vi "DROPBEAR_Model_Updating_Postprocessing.vi"(8 "error in (no error)":errorcluster, 11 "DROPBEAR_Model_Updating in":refnum<class "DROPBEAR_Model_Updating.lvclass">) -> (0 "Cycle time (ms)":dbl, 1 "Signal Quality":T3, 2 "Timing stats":T1, 3 "Plots":T2)   [LabVIEW 2021, in "DROPBEAR_Model_Updating.lvclass"]
uses:
  DROPBEAR_Model_Updating.lvclass
  DROPBEAR_Model_Updating.lvclass/DROPBEAR_Model_Updating.ctl
  Online_TRAC/Online_TRAC.lvclass/Online_TRAC.ctl
  Online_SNR/Online_SNR.lvclass/Online_SNR.ctl
  Read Distributional Statistics.vi
  Data_Array/Data_Array.lvclass
  Online_Statistic/Online_Statistic.lvclass
  Online_SNR/Online_SNR.lvclass
  Online_TRAC/Online_TRAC.lvclass
panel:
  out "Frequency":dynamicdata(graph)
  out "Nodal":dynamicdata(graph)
  out "Meter":dynamicdata(graph)
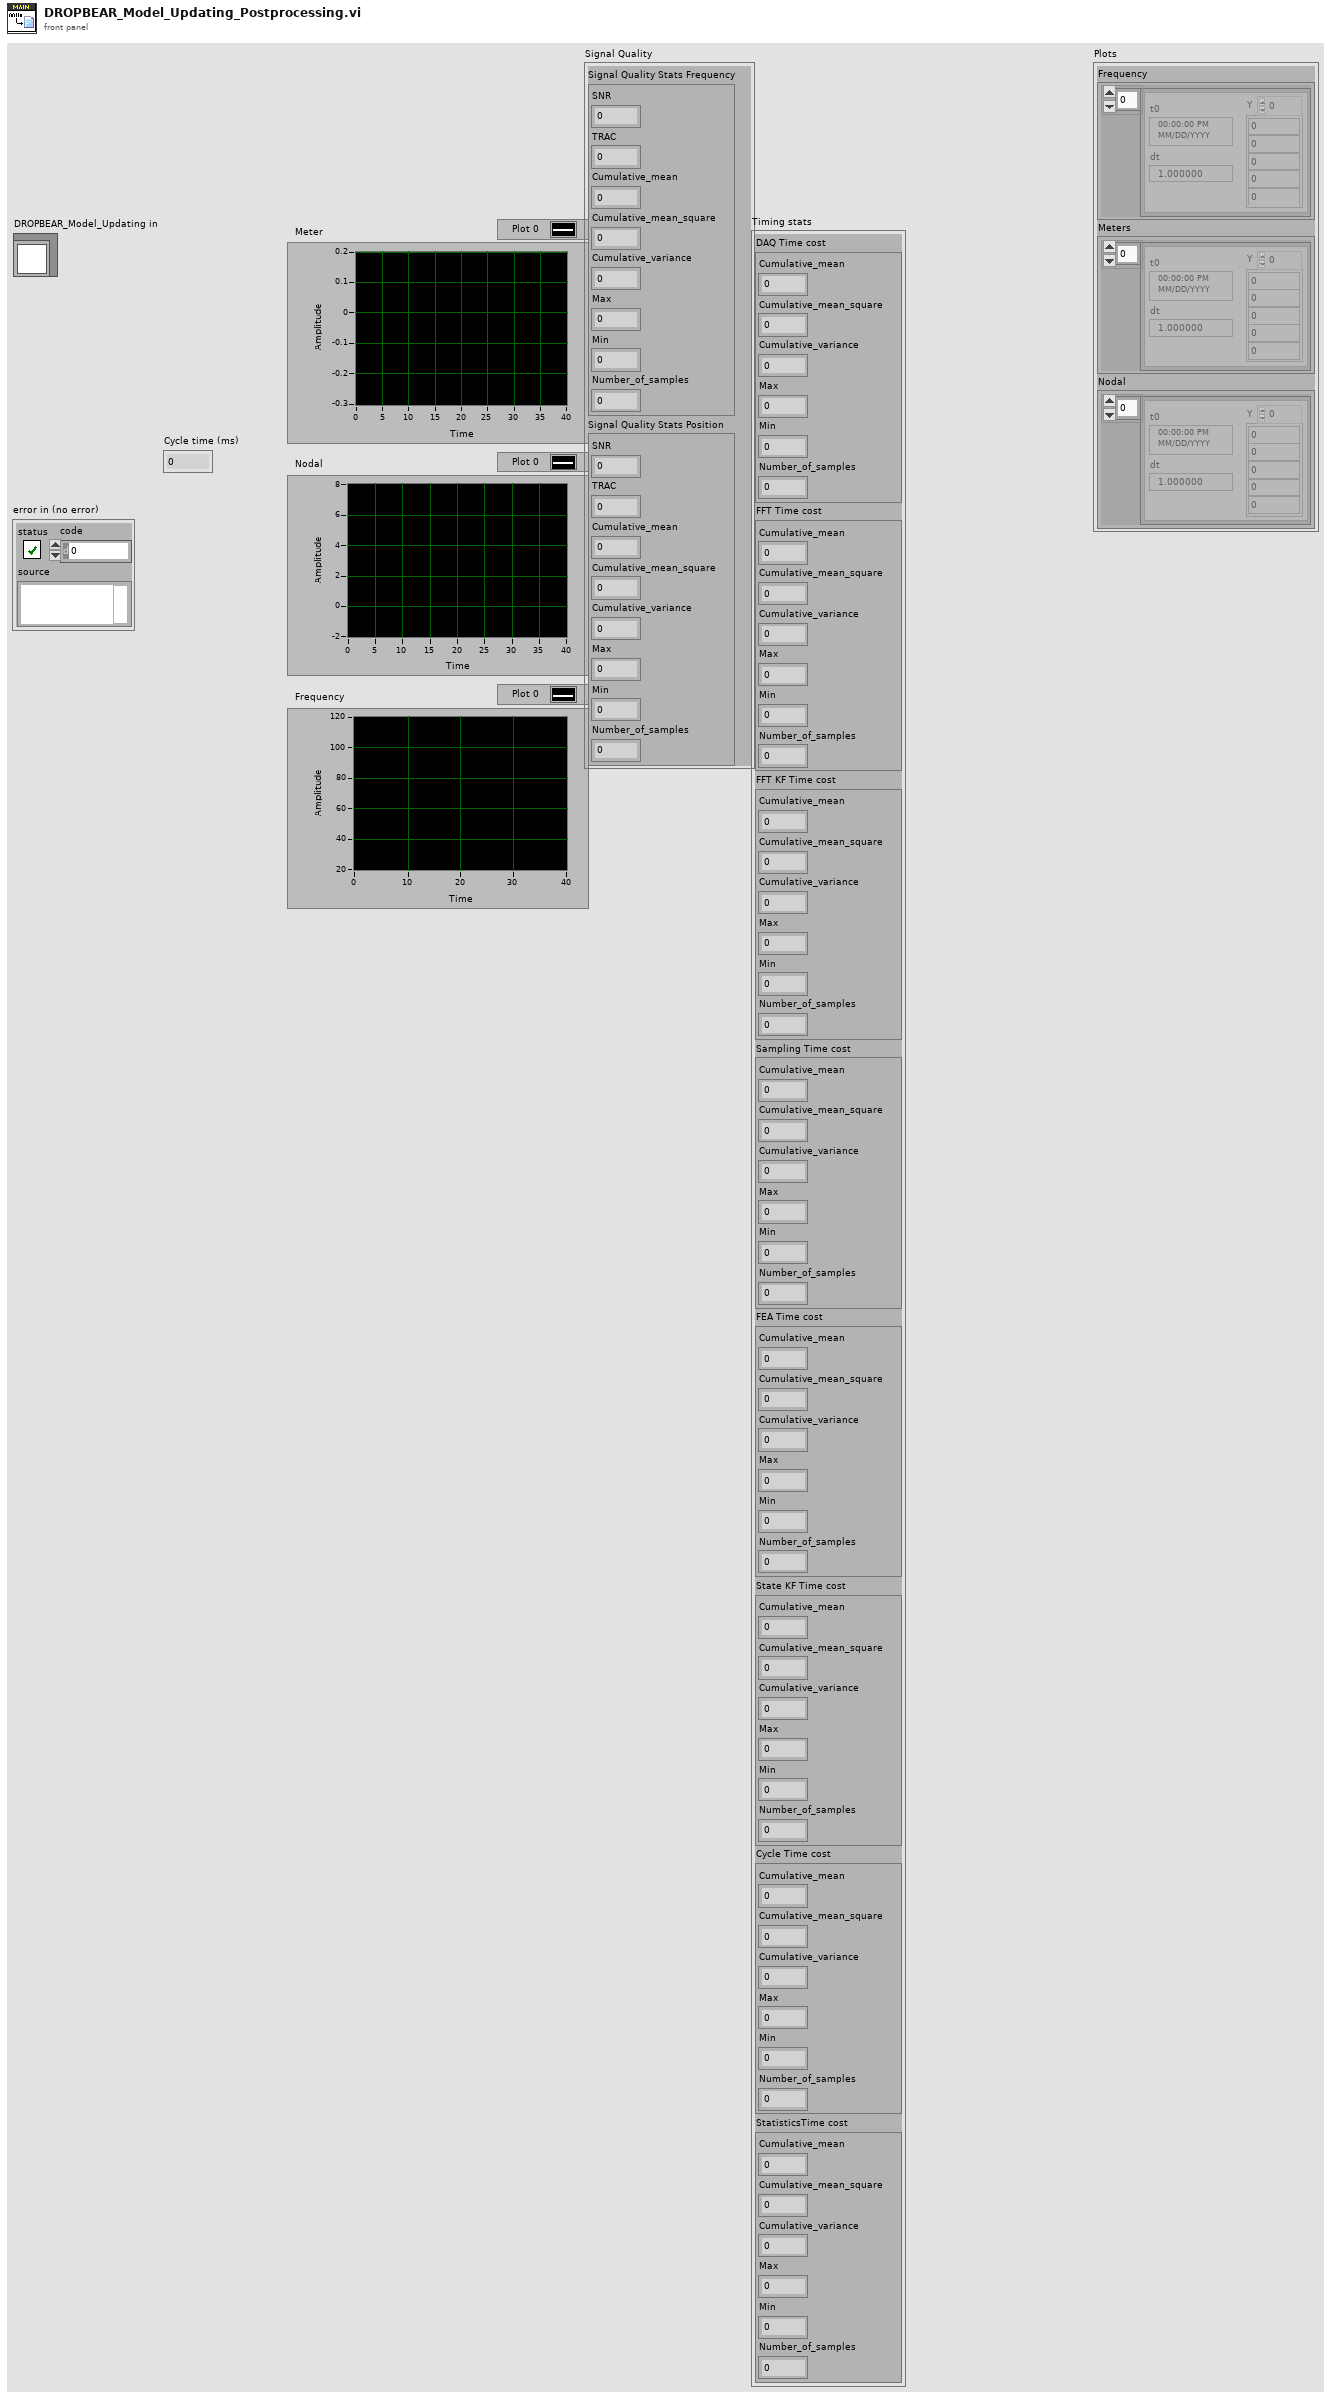
[diagram p1: front panel]
types:
  T1 = cluster{"DAQ Time cost":cluster{"Cumulative_mean":dbl, "Cumulative_mean_square ":dbl, "Cumulative_variance":dbl, "Max":dbl, "Min":dbl, "Number_of_samples":i32}, "FFT Time cost":cluster{"Cumulative_mean":dbl, "Cumulative_mean_square ":dbl, "Cumulative_variance":dbl, "Max":dbl, "Min":dbl, "Number_of_samples":i32}, "FFT KF Time cost":cluster{"Cumulative_mean":dbl, "Cumulative_mean_square ":dbl, "Cumulative_variance":dbl, "Max":dbl, "Min":dbl, "Number_of_samples":i32}, "Sampling Time cost":cluster{"Cumulative_mean":dbl, "Cumulative_mean_square ":dbl, "Cumulative_variance":dbl, "Max":dbl, "Min":dbl, "Number_of_samples":i32}, "FEA Time cost":cluster{"Cumulative_mean":dbl, "Cumulative_mean_square ":dbl, "Cumulative_variance":dbl, "Max":dbl, "Min":dbl, "Number_of_samples":i32}, "State KF Time cost":cluster{"Cumulative_mean":dbl, "Cumulative_mean_square ":dbl, "Cumulative_variance":dbl, "Max":dbl, "Min":dbl, "Number_of_samples":i32}, "Cycle Time cost":cluster{"Cumulative_mean":dbl, "Cumulative_mean_square ":dbl, "Cumulative_variance":dbl, "Max":dbl, "Min":dbl, "Number_of_samples":i32}, "StatisticsTime cost":cluster{"Cumulative_mean":dbl, "Cumulative_mean_square ":dbl, "Cumulative_variance":dbl, "Max":dbl, "Min":dbl, "Number_of_samples":i32}}
  T2 = cluster{"Frequency":dynamicdata, "Meters":dynamicdata, "Nodal":dynamicdata}
  T3 = cluster{"Signal Quality Stats Frequency":cluster{"SNR":dbl, "TRAC":dbl, "Cumulative_mean":dbl, "Cumulative_mean_square ":dbl, "Cumulative_variance":dbl, "Max":dbl, "Min":dbl, "Number_of_samples":i32}, "Signal Quality Stats Position":cluster{"SNR":dbl, "TRAC":dbl, "Cumulative_mean":dbl, "Cumulative_mean_square ":dbl, "Cumulative_variance":dbl, "Max":dbl, "Min":dbl, "Number_of_samples":i32}}
  T4 = cluster{"Displacement Measured Nodal ":refnum<class "Data_Array.lvclass">, "Displacement Measured Meters":refnum<class "Data_Array.lvclass">, "Displacement Estimate Nodal":refnum<class "Data_Array.lvclass">, "Displacement Estimate Meters":refnum<class "Data_Array.lvclass">, "Frequency Measured":refnum<class "Data_Array.lvclass">, "Frequency at Estimate":refnum<class "Data_Array.lvclass">}
  T5 = cluster{"Data Acquistion Time Cost":refnum<class "Online_Statistic.lvclass">, "FFT Time Cost":refnum<class "Online_Statistic.lvclass">, "Frequency Tracking Time Cost":refnum<class "Online_Statistic.lvclass">, "Sample Location Time Cost":refnum<class "Online_Statistic.lvclass">, "FEA Time Cost":refnum<class "Online_Statistic.lvclass">, "State Tracking Time Cost":refnum<class "Online_Statistic.lvclass">, "Online Cycle Time Cost":refnum<class "Online_Statistic.lvclass">, "Store Statistics Time Cost":refnum<class "Online_Statistic.lvclass">}
  T6 = cluster{"Cumulative_mean":dbl, "Cumulative_mean_square ":dbl, "Cumulative_variance":dbl, "Max":dbl, "Min":dbl, "Number_of_samples":i32}
  T7 = cluster{"SNR":dbl, "TRAC":dbl, "Cumulative_mean":dbl, "Cumulative_mean_square ":dbl, "Cumulative_variance":dbl, "Max":dbl, "Min":dbl, "Number_of_samples":i32}
  T8 = cluster{"Online_SNR_Frequency":refnum<class "Online_SNR.lvclass">, "Online_TRAC_Frequency":refnum<class "Online_TRAC.lvclass">, "Model_Error_Frequency":refnum<class "Online_Statistic.lvclass">, "Online_SNR_Position_Meters":refnum<class "Online_SNR.lvclass">, "Online_TRAC_Meters":refnum<class "Online_TRAC.lvclass">, "Model_Error_Meters":refnum<class "Online_Statistic.lvclass">}
  T9 = cluster{"Modeling Parameters input controls":cluster{"beam_length":dbl, "youngs_modulus":dbl, "torsion_spring":dbl, "beam_height":dbl, "beam_width":dbl, "beam_density":dbl, "number_of_FEA_nodes":i32, "accelerometer_mass":dbl}, "Mockbear input controls":cluster{"Dataset":string, "Resample Method":enum16{"Recorded", "Auto Resample", "Custom Resample"}}, "Simulation Parameters input controls":cluster{"Eigensolver ":enum16{"LabVIEW Cholesky", "LabVIEW General", "LabVIEW Inverse", "LEMP"}, "Models Forcasted":i32, "Max Roller Velocity":dbl, "Max Roller Position Percent":dbl, "Min Roller Position Percent":dbl}, "Program Controls":cluster{"Frequency KF":bool, "Pinned State KF":bool, "FFT Bounding":bool, "Filter Constants Frequency":cluster{"Measurement Variance":dbl, "State Variance":dbl, "Threshold":dbl}, "Filter Constants Position":cluster{"Measurement Variance":dbl, "State Variance":dbl, "Threshold":dbl}, "Moving Window Size":i32, "Time Series buffer":dbl, "Record Time Series Data":bool, "Record Moving Window Data":bool, "Record Online Error Metrics ":bool, "Record Statistics":bool}}
  T10 = enum16{"LabVIEW Cholesky", "LabVIEW General", "LabVIEW Inverse", "LEMP"}
  T11 = enum16{"Recorded", "Auto Resample", "Custom Resample"}
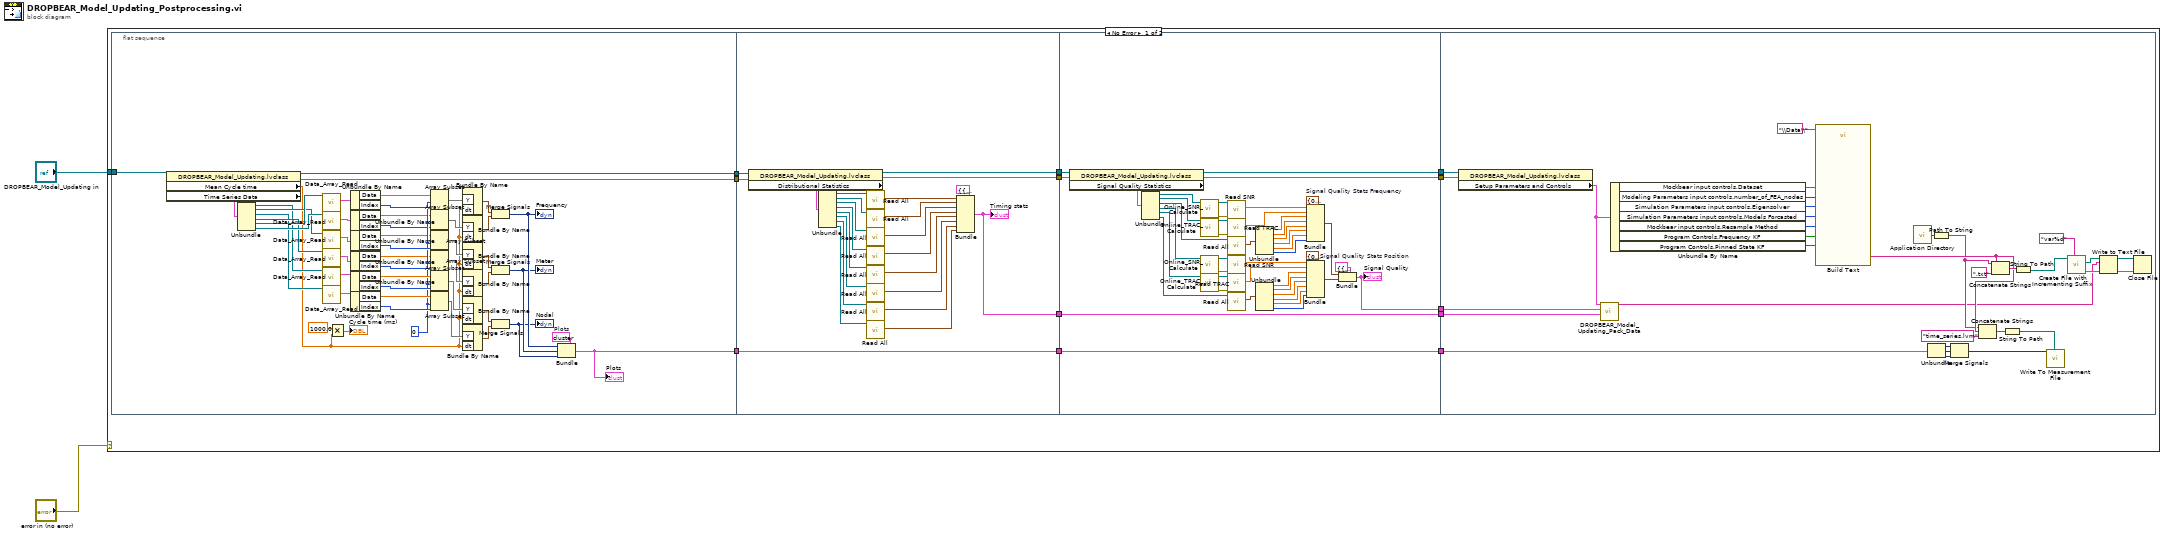
[diagram p0: block diagram]
diagram:
  n1 = case shown="No Error" "error in (no error)" {
    tunnel: "DROPBEAR_Model_Updating in" -> [w15 _]
    frame No Error {
      n2 = flat-sequence {
        tunnel: w15 -> [w23]
        tunnel: [w22] -> w10
        tunnel: [w21] -> w9
        tunnel: [w16] -> w6
        tunnel: [w71] -> w14
        tunnel: [w70] -> w13
        tunnel: w10 -> [w69]
        tunnel: w9 -> [w68]
        tunnel: [w66] -> w8
        tunnel: [w65] -> w7
        tunnel: w6 -> [w65]
        tunnel: w14 -> [w133]
        tunnel: w13 -> [w132]
        tunnel: [w98] -> w12
        tunnel: [w97] -> w11
        tunnel: w8 -> [w89]
        tunnel: w7 -> [w91]
        tunnel: [w91] -> w5
        tunnel: [w90] -> w4
        tunnel: [w89] -> w3
        tunnel: w12 -> [w161]
        tunnel: w11 -> [w160]
        tunnel: w5 -> [w165]
        tunnel: w4 -> [w135]
        tunnel: w3 -> [w134]
        frame #0 {
          w17 = T2 {"Frequency"=[], "Meters"=[], "Nodal"=[]}  # Plots
          w51 = 0 ("index")
          n3 = property class="DROPBEAR_Model_Updating.lvclass"(reference=w23) -> (reference out=w22:refnum<class "DROPBEAR_Model_Updating.lvclass">, error out=w21:errorcluster, "Mean Cycle time"=w24:dbl, "Time Series Data"=w31:T4)  [unwired: 1 in]
          n4 = Unbundle(w31) -> ("Displacement Measured Nodal"=w26:refnum<class "Data_Array.lvclass">, "Displacement Measured Meters"=w28:refnum<class "Data_Array.lvclass">, "Displacement Estimate Nodal"=w25:refnum<class "Data_Array.lvclass">, "Displacement Estimate Meters"=w27:refnum<class "Data_Array.lvclass">, "Frequency Measured"=w30:refnum<class "Data_Array.lvclass">, "Frequency at Estimate"=w29:refnum<class "Data_Array.lvclass">)
          n5 = call-dynamic "Data_Array_Read.vi"("Data_Array in"=w30) -> ("Data_params"=w49:cluster{"Data":dbl[], "Index":i32, "Buffer":i32})  [unwired: 8 in, 2 out]
          n6 = call-dynamic "Data_Array_Read.vi"("Data_Array in"=w29) -> ("Data_params"=w50:cluster{"Data":dbl[], "Index":i32, "Buffer":i32})  [unwired: 8 in, 2 out]
          n7 = call-dynamic "Data_Array_Read.vi"("Data_Array in"=w28) -> ("Data_params"=w56:cluster{"Data":dbl[], "Index":i32, "Buffer":i32})  [unwired: 8 in, 2 out]
          n8 = call-dynamic "Data_Array_Read.vi"("Data_Array in"=w27) -> ("Data_params"=w55:cluster{"Data":dbl[], "Index":i32, "Buffer":i32})  [unwired: 8 in, 2 out]
          n9 = call-dynamic "Data_Array_Read.vi"("Data_Array in"=w26) -> ("Data_params"=w59:cluster{"Data":dbl[], "Index":i32, "Buffer":i32})  [unwired: 8 in, 2 out]
          n10 = call-dynamic "Data_Array_Read.vi"("Data_Array in"=w25) -> ("Data_params"=w60:cluster{"Data":dbl[], "Index":i32, "Buffer":i32})  [unwired: 8 in, 2 out]
          n11 = Multiply(x=1000.0, y=w24) -> (x*y=→"Cycle time (ms)":dbl)
          n12 = Unbundle By Name(w49) -> ("Data"=w47:dbl[], "Index"=w52:i32)
          n13 = Unbundle By Name(w50) -> ("Data"=w46:dbl[], "Index"=w48:i32)
          n14 = Unbundle By Name(w56) -> ("Data"=w45:dbl[], "Index"=w58:i32)
          n15 = Unbundle By Name(w55) -> ("Data"=w44:dbl[], "Index"=w57:i32)
          n16 = Unbundle By Name(w59) -> ("Data"=w62:dbl[], "Index"=w64:i32)
          n17 = Unbundle By Name(w60) -> ("Data"=w61:dbl[], "Index"=w63:i32)
          n18 = Array Subset(array=w47, index=w51, length=w52) -> (w43:dbl[])
          n19 = Array Subset(array=w46, index=w51, length=w48) -> (w42:dbl[])
          n20 = Array Subset(array=w45, index=w51, length=w58) -> (w41:dbl[])
          n21 = Array Subset(array=w44, index=w51, length=w57) -> (w40:dbl[])
          n22 = Array Subset(array=w62, index=w51, length=w64) -> (w39:dbl[])
          n23 = Array Subset(array=w61, index=w51, length=w63) -> (w38:dbl[])
          n24 = Bundle By Name("Y"=w43, "dt"=w24) -> (w37:waveform(dbl))  [unwired: 1 in]
          n25 = Bundle By Name("Y"=w42, "dt"=w24) -> (w36:waveform(dbl))  [unwired: 1 in]
          n26 = Bundle By Name("Y"=w41, "dt"=w24) -> (w35:waveform(dbl))  [unwired: 1 in]
          n27 = Bundle By Name("Y"=w40, "dt"=w24) -> (w34:waveform(dbl))  [unwired: 1 in]
          n28 = Bundle By Name("Y"=w39, "dt"=w24) -> (w33:waveform(dbl))  [unwired: 1 in]
          n29 = Bundle By Name("Y"=w38, "dt"=w24) -> (w32:waveform(dbl))  [unwired: 1 in]
          n30 = Merge Signals(w37, w36) -> (w20:dynamicdata)
          "Frequency" <- w20
          n31 = Merge Signals(w35, w34) -> (w19:dynamicdata)
          "Meter" <- w19
          n32 = Merge Signals(w33, w32) -> (w18:dynamicdata)
          "Nodal" <- w18
          n33 = Bundle(cluster=w17, "Frequency"=w20, "Meters"=w19, "Nodal"=w18) -> (w16:T2)
          "Plots" <- w16
        }
        frame #1 {
          n34 = property class="DROPBEAR_Model_Updating.lvclass"(reference=w69, error in=w68) -> (reference out=w71:refnum<class "DROPBEAR_Model_Updating.lvclass">, error out=w70:errorcluster, "Distributional Statistics"=w88:T5)
          n35 = Unbundle(w88) -> ("Data Acquistion Time Cost"=w87:refnum<class "Online_Statistic.lvclass">, "FFT Time Cost"=w86:refnum<class "Online_Statistic.lvclass">, "Frequency Tracking Time Cost"=w85:refnum<class "Online_Statistic.lvclass">, "Sample Location Time Cost"=w84:refnum<class "Online_Statistic.lvclass">, "FEA Time Cost"=w83:refnum<class "Online_Statistic.lvclass">, "State Tracking Time Cost"=w82:refnum<class "Online_Statistic.lvclass">, "Online Cycle Time Cost"=w81:refnum<class "Online_Statistic.lvclass">, "Store Statistics Time Cost"=w80:refnum<class "Online_Statistic.lvclass">)
          n36 = call "Read All.vi"("Online_Statistic in"=w87) -> ("Statistics"=w79:T6)  [unwired: 8 in, 2 out]
          n37 = call "Read All.vi"("Online_Statistic in"=w86) -> ("Statistics"=w78:T6)  [unwired: 8 in, 2 out]
          n38 = call "Read All.vi"("Online_Statistic in"=w85) -> ("Statistics"=w77:T6)  [unwired: 8 in, 2 out]
          n39 = call "Read All.vi"("Online_Statistic in"=w84) -> ("Statistics"=w76:T6)  [unwired: 8 in, 2 out]
          n40 = call "Read All.vi"("Online_Statistic in"=w83) -> ("Statistics"=w75:T6)  [unwired: 8 in, 2 out]
          n41 = call "Read All.vi"("Online_Statistic in"=w82) -> ("Statistics"=w74:T6)  [unwired: 8 in, 2 out]
          n42 = call "Read All.vi"("Online_Statistic in"=w81) -> ("Statistics"=w73:T6)  [unwired: 8 in, 2 out]
          n43 = call "Read All.vi"("Online_Statistic in"=w80) -> ("Statistics"=w72:T6)  [unwired: 8 in, 2 out]
          n44 = Bundle(cluster=T1 {"DAQ Time cost"={"Cumulative_mean"=0.0, "Cumulative_mean_square "=0.0, "Cumulative_variance"=0.0, "Max"=0.0, "Min"=0.0, "Number_of_samples"=0}, "FFT Time cost"={"Cumulative_mean"=0.0, "Cumulative_mean_square "=0.0, "Cumulative_variance"=0.0, "Max"=0.0, "Min"=0.0, "Number_of_samples"=0}, "FFT KF Time cost"={"Cumulative_mean"=0.0, "Cumulative_mean_square "=0.0, "Cumulative_variance"=0.0, "Max"=0.0, "Min"=0.0, "Number_of_samples"=0}, "Sampling Time cost"={"Cumulative_mean"=0.0, "Cumulative_mean_square "=0.0, "Cumulative_variance"=0.0, "Max"=0.0, "Min"=0.0, "Number_of_samples"=0}, "FEA Time cost"={"Cumulative_mean"=0.0, "Cumulative_mean_square "=0.0, "Cumulative_variance"=0.0, "Max"=0.0, "Min"=0.0, "Number_of_samples"=0}, "State KF Time cost"={"Cumulative_mean"=0.0, "Cumulative_mean_square "=0.0, "Cumulative_variance"=0.0, "Max"=0.0, "Min"=0.0, "Number_of_samples"=0}, "Cycle Time cost"={"Cumulative_mean"=0.0, "Cumulative_mean_square "=0.0, "Cumulative_variance"=0.0, "Max"=0.0, "Min"=0.0, "Number_of_samples"=0}, "StatisticsTime cost"={"Cumulative_mean"=0.0, "Cumulative_mean_square "=0.0, "Cumulative_variance"=0.0, "Max"=0.0, "Min"=0.0, "Number_of_samples"=0}} ("Timing stats"), "DAQ Time cost"=w79, "FFT Time cost"=w78, "FFT KF Time cost"=w77, "Sampling Time cost"=w76, "FEA Time cost"=w75, "State KF Time cost"=w74, "Cycle Time cost"=w73, "StatisticsTime cost"=w72) -> (w66:T1)
          "Timing stats" <- w66
        }
        frame #2 {
          w95 = T7 {"SNR"=0.0, "TRAC"=0.0, "Cumulative_mean"=0.0, "Cumulative_mean_square "=0.0, "Cumulative_variance"=0.0, "Max"=0.0, "Min"=0.0, "Number_of_samples"=0}  # Signal Quality Stats Frequency
          w96 = T7 {"SNR"=0.0, "TRAC"=0.0, "Cumulative_mean"=0.0, "Cumulative_mean_square "=0.0, "Cumulative_variance"=0.0, "Max"=0.0, "Min"=0.0, "Number_of_samples"=0}  # Signal Quality Stats Position
          n45 = property class="DROPBEAR_Model_Updating.lvclass"(reference=w133, error in=w132) -> (reference out=w98:refnum<class "DROPBEAR_Model_Updating.lvclass">, error out=w97:errorcluster, "Signal Quality Statistics"=w131:T8)
          n46 = Unbundle(w131) -> ("Online_SNR_Frequency"=w130:refnum<class "Online_SNR.lvclass">, "Online_TRAC_Frequency"=w129:refnum<class "Online_TRAC.lvclass">, "Model_Error_Frequency"=w126:refnum<class "Online_Statistic.lvclass">, "Online_SNR_Position_Meters"=w128:refnum<class "Online_SNR.lvclass">, "Online_TRAC_Meters"=w127:refnum<class "Online_TRAC.lvclass">, "Model_Error_Meters"=w125:refnum<class "Online_Statistic.lvclass">)
          n47 = call "Online_SNR_Calculate.vi"("Online_SNR in"=w130) -> ("error out"=w121:errorcluster, "Online_SNR out"=w122:refnum<class "Online_SNR.lvclass">)  [unwired: 9 in]
          n48 = call "Online_TRAC_Calculate.vi"("Online_TRAC in"=w129) -> ("error out"=w120:errorcluster, "Online_TRAC out"=w119:refnum<class "Online_TRAC.lvclass">)  [unwired: 9 in]
          n49 = call "Online_SNR_Calculate.vi"("Online_SNR in"=w128) -> ("error out"=w124:errorcluster, "Online_SNR out"=w123:refnum<class "Online_SNR.lvclass">)  [unwired: 9 in]
          n50 = call "Online_TRAC_Calculate.vi"("Online_TRAC in"=w127) -> ("error out"=w118:errorcluster, "Online_TRAC out"=w117:refnum<class "Online_TRAC.lvclass">)  [unwired: 9 in]
          n51 = call "Read SNR.vi"("error in (no error)"=w121, "Online_SNR in"=w122) -> ("SNR"=w116:dbl)  [unwired: 7 in, 2 out]
          n52 = call "Read TRAC.vi"("error in (no error)"=w120, "Online_TRAC in"=w119) -> ("TRAC"=w115:dbl)  [unwired: 7 in, 2 out]
          n53 = call "Read All.vi"("Online_Statistic in"=w126) -> ("Statistics"=w114:T6)  [unwired: 8 in, 2 out]
          n54 = call "Read SNR.vi"("error in (no error)"=w124, "Online_SNR in"=w123) -> ("SNR"=w106:dbl)  [unwired: 7 in, 2 out]
          n55 = call "Read TRAC.vi"("error in (no error)"=w118, "Online_TRAC in"=w117) -> ("TRAC"=w105:dbl)  [unwired: 7 in, 2 out]
          n56 = call "Read All.vi"("Online_Statistic in"=w125) -> ("Statistics"=w107:T6)  [unwired: 8 in, 2 out]
          n57 = Unbundle(w114) -> ("Cumulative_mean"=w113:dbl, "Cumulative_mean_square"=w112:dbl, "Cumulative_variance"=w111:dbl, "Max"=w110:dbl, "Min"=w109:dbl, "Number_of_samples"=w108:i32)
          n58 = Unbundle(w107) -> ("Cumulative_mean"=w104:dbl, "Cumulative_mean_square"=w103:dbl, "Cumulative_variance"=w102:dbl, "Max"=w101:dbl, "Min"=w100:dbl, "Number_of_samples"=w99:i32)
          n59 = Bundle(cluster=w95, "SNR"=w116, "TRAC"=w115, "Cumulative_mean"=w113, "Cumulative_mean_square"=w112, "Cumulative_variance"=w111, "Max"=w110, "Min"=w109, "Number_of_samples"=w108) -> (w94:T7)
          n60 = Bundle(cluster=w96, "SNR"=w106, "TRAC"=w105, "Cumulative_mean"=w104, "Cumulative_mean_square"=w103, "Cumulative_variance"=w102, "Max"=w101, "Min"=w100, "Number_of_samples"=w99) -> (w93:T7)
          n61 = Bundle(cluster=T3 {"Signal Quality Stats Frequency"={"SNR"=0.0, "TRAC"=0.0, "Cumulative_mean"=0.0, "Cumulative_mean_square "=0.0, "Cumulative_variance"=0.0, "Max"=0.0, "Min"=0.0, "Number_of_samples"=0}, "Signal Quality Stats Position"={"SNR"=0.0, "TRAC"=0.0, "Cumulative_mean"=0.0, "Cumulative_mean_square "=0.0, "Cumulative_variance"=0.0, "Max"=0.0, "Min"=0.0, "Number_of_samples"=0}}, "Signal Quality Stats Frequency"=w94, "Signal Quality Stats Position"=w93) -> (w90:T3)
          "Signal Quality" <- w90
        }
        frame #3 {
          n62 = property class="DROPBEAR_Model_Updating.lvclass"(reference=w161, error in=w160) -> ("Setup Parameters and Controls"=w136:T9)  [unwired: 2 out]
          n63 = call "DROPBEAR_Model_Updating_Pack_Data.vi"("Timing stats"=w134, "Signal Quality"=w135, "Setup Parameters and Controls"=w136) -> ("String"=w137:string)  [unwired: 8 in]
          n64 = Unbundle By Name(w136) -> ("Mockbear input controls.Dataset"=w159:string, "Modeling Parameters input controls.number_of_FEA_nodes"=w158:i32, "Simulation Parameters input controls.Eigensolver"=w157:T10, "Simulation Parameters input controls.Models Forcasted"=w156:i32, "Mockbear input controls.Resample Method"=w155:T11, "Program Controls.Frequency KF"=w154:bool, "Program Controls.Pinned State KF"=w153:bool)
          n65 = call "Build Text"("Beginning Text"="\\Data\\", "models"=w156, "kf_freq"=w154, "dataset"=w159, "nodes"=w158, "eigensolver"=w157, "sampling"=w155, "kf_fea"=w153) -> ("Result"=w144:string)  [unwired: 6 in, 1 out]
          n66 = call <vilib>:"Application Directory.vi"() -> ("Application Directory"=w143:path)
          n67 = Unbundle(w165) -> ("Frequency"=w164:dynamicdata, "Meters"=w163:dynamicdata, "Nodal"=w162:dynamicdata)
          n68 = Path To String(path=w143) -> (string=w140:string)
          n69 = Merge Signals(w164, w163, w162) -> (w166:dynamicdata)
          n70 = Concatenate Strings(w140, w144, "time_series.lvm" ("string")) -> (w142:string)
          n71 = Concatenate Strings(w140, w144, ".txt" ("string")) -> (w146:string)
          n72 = String To Path(string=w142) -> (path=w141:path)
          n73 = String To Path(string=w146) -> (path=w139:path)
          n74 = call "Write To Measurement File"("Signals"=w166, "Filename"=w141) -> ()  [unwired: 15 in, 3 out]
          n75 = call <vilib>:"Create File with Incrementing Suffix.vi"("format string (\" (%d)\")"="var%d" ("string"), "file path"=w139) -> ("error out"=w151:errorcluster, "actual path"=w150:path)  [unwired: 7 in, 1 out]
          n76 = Write to Text File(file (use dialog)=w150, text=w137, error in=w151) -> (refnum out=w149:refnum<file>, error out=w148:errorcluster)  [unwired: 1 in, 1 out]
          n77 = Close File(refnum=w149, error in=w148) -> ()  [unwired: 2 out]
        }
      }
    }
    frame Error {
    }
  }
